vi "Parse Results (table).vi"(8 "error in (no error)":errorcluster, 11 "Results.Results (Dictionary)":cluster{"key":string, "value":dbl}[](array[cluster])) -> (0 "error out":errorcluster, 2 "Table Control":string[][](table), 3 "Results (Dictionary)":cluster{"key":string, "value":dbl}[](array[cluster]))   [LabVIEW 2016, in "Instrument.Lockin.lvclass"]
uses:
  Instrument.Lockin.lvclass
  Typedefs/Results Type--Enum.ctl
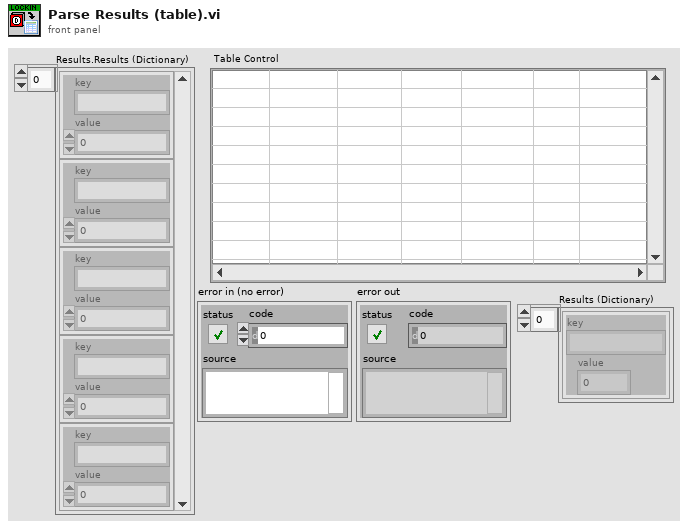
[diagram p1: front panel]
types:
  T1 = typedef "Instrument.Lockin.lvclass/Results Type--Enum.ctl" = enum16{"X", "Y", "R", "Theta", "Mean"}
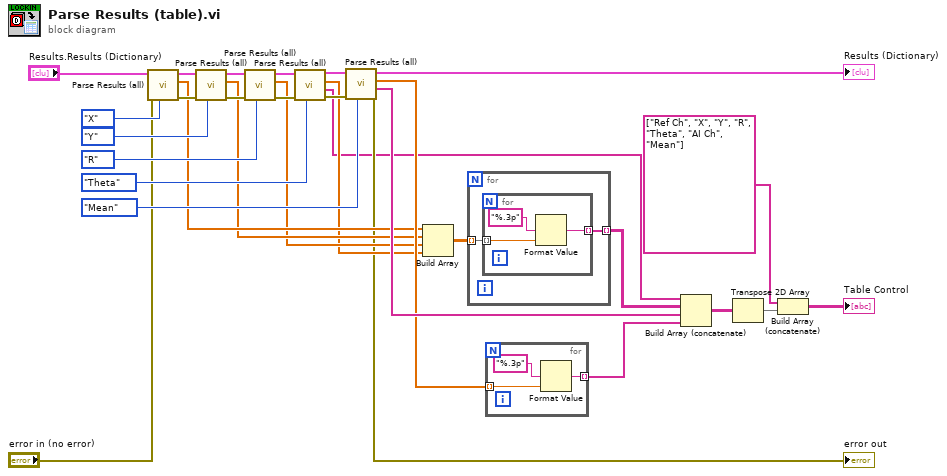
[diagram p0: block diagram]
diagram:
  n1 = call "Parse Results (all).vi"("Type"=Results_Type--Enum."X", "error in (no error)"="error in (no error)", "Results (Dictionary)"="Results.Results (Dictionary)") -> ("error out"=w30:errorcluster, "Data"=w8:dbl[], "Results (Dictionary)"=w29:cluster{"key":string, "value":dbl}[])  [unwired: 5 in, 1 out]
  n2 = call "Parse Results (all).vi"("Type"=Results_Type--Enum."Y", "error in (no error)"=w30, "Results (Dictionary)"=w29) -> ("error out"=w28:errorcluster, "Data"=w7:dbl[], "Results (Dictionary)"=w27:cluster{"key":string, "value":dbl}[])  [unwired: 5 in, 1 out]
  n3 = call "Parse Results (all).vi"("Type"=Results_Type--Enum."R", "error in (no error)"=w28, "Results (Dictionary)"=w27) -> ("error out"=w23:errorcluster, "Data"=w6:dbl[], "Results (Dictionary)"=w24:cluster{"key":string, "value":dbl}[])  [unwired: 5 in, 1 out]
  n4 = call "Parse Results (all).vi"("Type"=Results_Type--Enum."Theta", "error in (no error)"=w23, "Results (Dictionary)"=w24) -> ("error out"=w26:errorcluster, "Names"=w2:string[], "Data"=w5:dbl[], "Results (Dictionary)"=w25:cluster{"key":string, "value":dbl}[])  [unwired: 5 in]
  n5 = call "Parse Results (all).vi"("Type"=Results_Type--Enum."Mean", "error in (no error)"=w26, "Results (Dictionary)"=w25) -> ("error out"=→"error out":errorcluster, "Names"=w17:string[], "Data"=w11:dbl[], "Results (Dictionary)"=→"Results (Dictionary)":cluster{"key":string, "value":dbl}[])  [unwired: 5 in]
  n6 = Build Array(w8, w7, w6, w5) -> (w12:dbl[][])
  n7 = for {
    tunnel: [w33] -> w3 mode=indexing
    tunnel: w12 -> [w32] mode=indexing
    n8 = for {
      tunnel: [w36] -> w33 mode=indexing
      tunnel: w32 -> [w35] mode=indexing
      n9 = Format Value(format string="%.3p", value (0)=w35) -> (output string=w36:string)  [unwired: 1 in]
    }
  }
  n10 = for {
    tunnel: w11 -> [w38] mode=indexing
    tunnel: [w37] -> w1 mode=indexing
    n11 = Format Value(format string="%.3p", value (0)=w38) -> (output string=w37:string)  [unwired: 1 in]
  }
  n12 = Build Array (concatenate)(w2, w3, w17, w1) -> (w16:string[][])
  n13 = Transpose 2D Array(2D array=w16) -> (transposed array=w15:string[][])
  n14 = Build Array (concatenate)(string[] ["Ref Ch", "X", "Y", "R", "Theta", "AI Ch", "Mean"] ("Names"), w15) -> (→"Table Control":string[][])
